vi "S2C_Access_CreateTable.vi"(8 "Error In":errorcluster) -> (0 "Error Out":errorcluster, 2 "Canceled?":bool, 3 "TableName":string)   [LabVIEW 2015]
uses:
  S2C_Access_Globals.vi
  <vilib>/addons/database/Connection.llb/Conn Execute.vi
  <vilib>/addons/database/Recordset.llb/Rec Destroy - Connection.vi
  <vilib>/addons/database/NI_Database_API.lvlib
panel:
  out "Init":bool
  in  "Create":bool
  in  "Table":string caption="Table Name"
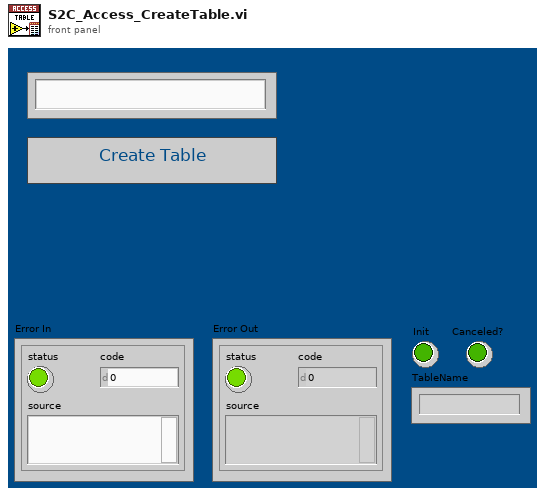
[diagram p1: front panel]
types:
  T1 = typedef "NI_Database_API.lvlib/Conn ObjectReference.ctl" = refnum<k1>
  T2 = typedef "NI_Database_API.lvlib/Rec ObjectReference.ctl" = refnum<k1>
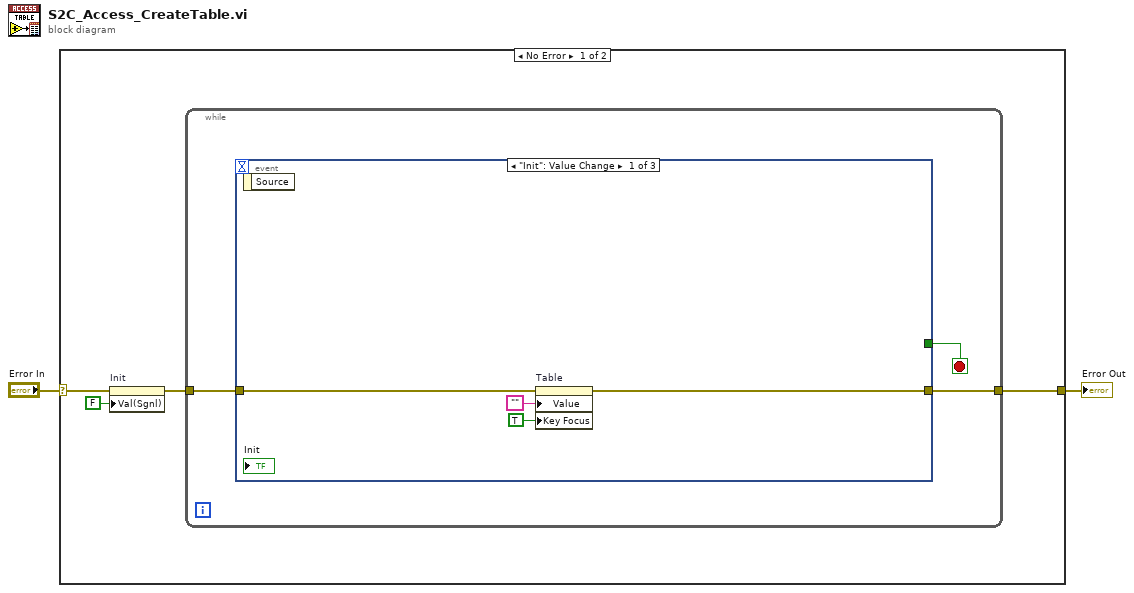
[diagram p0: block diagram]
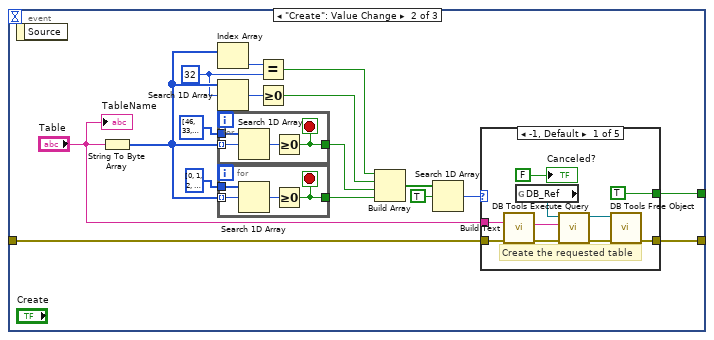
[diagram p2: hidden frame]
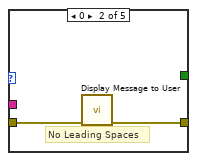
[diagram p3: hidden frame]
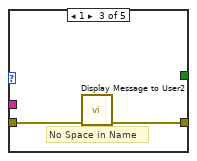
[diagram p4: hidden frame]
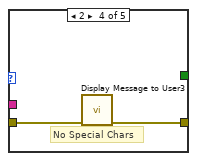
[diagram p5: hidden frame]
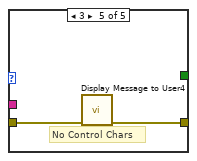
[diagram p6: hidden frame]
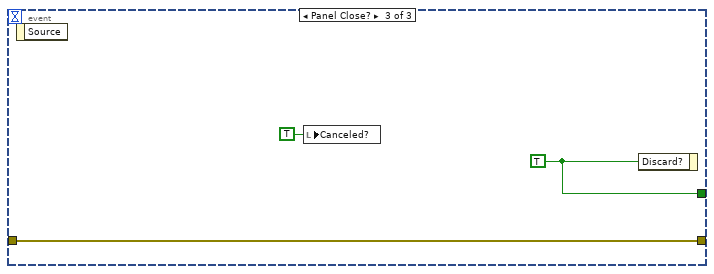
[diagram p7: hidden frame]
diagram:
  n1 = case shown="No Error" "Error In" {
    selector: "Error In" -> [w6 w60]
    tunnel: [w3 w60] -> w1
    frame No Error {
      n2 = property on="Init" class="Bool (strict)"(error in=w6, "Val(Sgnl)"=FALSE ("Value (Signaling)")) -> (error out=w5:errorcluster)  [unwired: 1 in, 1 out]
      n3 = while {
        tunnel: w5 -> [w9]
        tunnel: [w8] -> w3
        stop <- w7 stop-if-true
        n4 = event shown="[0] \"Init\": Value Change" {
          selector: _ -> [_ _ _]
          dyn-events: _ -> [_ _ _]
          timeout: _ -> [_ _ _]
          tunnel: w9 -> [w13 w17 w59]
          tunnel: [w10 w16 w59] -> w8
          tunnel: [_ w15 w58] -> w7
          event "Init": Value Change {
            n5 = event-data() -> ()  [unwired: 1 in, 1 out]
            n6 = property on="Table" class="Str"(error in=w13, "Value"="", "Key Focus"=TRUE) -> (error out=w10:errorcluster)  [unwired: 1 in, 1 out]
          }
          event "Create": Value Change {
            w20 = u8 32 ("element")
            n7 = event-data() -> ()  [unwired: 1 in, 1 out]
            n8 = String To Byte Array(string="Table") -> (unsigned byte array=w25:u8[])
            n9 = Index Array(array=w25) -> (element=w26:u8)  [unwired: 1 in]
            n10 = Search 1D Array(1D array=w25, element=w20) -> (index of element=w24:i32)  [unwired: 1 in]
            n11 = for {
              tunnel: u8[] [46, 33, 96, 91, 93, 34] -> [w56]
              tunnel: w25 -> [w55] mode=indexing
              tunnel: [w53] -> w29
              stop <- w53 stop-if-true
              n12 = Search 1D Array(1D array=w56, element=w55) -> (index of element=w54:i32)  [unwired: 1 in]
              n13 = Greater Or Equal To 0?(x=w54) -> (x >= 0?=w53:bool)
            }
            n14 = for {
              tunnel: u8[] [0, 1, 2, 3, 4, 5, 6, 7, 8, 9, 10, 11, 12, 13, 14, 15, 16, 17, 18, 19, 20, 21, 22, 23, 24, 25, 26, 27, 28, 29, 30, 31] ("Array") -> [w52]
              tunnel: w25 -> [w51] mode=indexing
              tunnel: [w49] -> w27
              stop <- w49 stop-if-true
              n15 = Search 1D Array(1D array=w52, element=w51) -> (index of element=w50:i32)  [unwired: 1 in]
              n16 = Greater Or Equal To 0?(x=w50) -> (x >= 0?=w49:bool)
            }
            n17 = Equal?(x=w26, y=w20) -> (x = y?=w19:bool)
            n18 = Greater Or Equal To 0?(x=w24) -> (x >= 0?=w18:bool)
            n19 = Build Array(w19, w18, w29, w27) -> (w23:bool[])
            n20 = Search 1D Array(1D array=w23, element=TRUE) -> (index of element=w21:i32)  [unwired: 1 in]
            n21 = case shown="-1, Default" w21 {
              tunnel: w17 -> [w33 w42 w44 w46 w48]
              tunnel: [w32 w41 w43 w45 w47] -> w16
              tunnel: [TRUE _ _ _ _] -> w15
              tunnel: "Table" -> [w31 _ _ _ _]
              frame -1, Default {
                # "Create the requested table"
                n22 = call "Build Text"("Table"=w31, "error in (no error)"=w33) -> ("Result"=w36:string, "error out"=w34:errorcluster)  [unwired: 12 in]
                n23 = global read "S2C_Access_Globals.vi" "DB_Ref"() -> (w35:T1)
                n24 = call-poly <vilib>:"DB Tools Execute Query.vi"("error in (no error)"=w34, "SQL query"=w36, "connection reference"=w35) -> ("error out"=w37:errorcluster, "recordset reference"=w38:T2)  [unwired: 5 in]
                n25 = call-poly <vilib>:"DB Tools Free Object.vi"("error in (no error)"=w37, "recordset reference"=w38) -> ("error out"=w32:errorcluster)  [unwired: 8 in, 1 out]
                "Canceled?" <- FALSE ("Canceled?")
              }
              frame 0 {
                # "No Leading Spaces"
                n26 = call "Display Message to User"("error in (no error)"=w42) -> ("error out"=w41:errorcluster)  [unwired: 9 in, 1 out]
              }
              frame 1 {
                # "No Space in Name"
                n27 = call "Display Message to User2"("error in (no error)"=w44) -> ("error out"=w43:errorcluster)  [unwired: 9 in, 1 out]
              }
              frame 2 {
                # "No Special Chars"
                n28 = call "Display Message to User3"("error in (no error)"=w46) -> ("error out"=w45:errorcluster)  [unwired: 9 in, 1 out]
              }
              frame 3 {
                # "No Control Chars"
                n29 = call "Display Message to User4"("error in (no error)"=w48) -> ("error out"=w47:errorcluster)  [unwired: 9 in, 1 out]
              }
            }
            "TableName" <- "Table"
          }
          event Panel Close? {
            w58 = TRUE ("Discard?")
            n30 = event-data() -> ()  [unwired: 1 in, 1 out]
            n31 = local write "Canceled?"(TRUE ("Canceled?")) -> ()
            n32 = event-data("Discard?"=w58) -> ()  [unwired: 1 in, 1 out]
          }
        }
      }
    }
    frame Error {
    }
  }
  "Error Out" <- w1
